vi "stirap_detect.vi"() -> ()   [LabVIEW 2012]
uses:
  <vilib>/DAQmx/create/channels.llb/DAQmx Create Channel (CO-Pulse Generation-Frequency).vi
  <vilib>/DAQmx/configure/timing.llb/DAQmx Timing (Implicit).vi
  <vilib>/Analysis/baseanly.llb/Mean (DBL).vi
  <vilib>/Utility/file.llb/Write To Spreadsheet File (DBL).vi
  <vilib>/Analysis/NI_AALBase.lvlib
panel:
  out "Fluorescence\n Mean Before":dbl format="%0.2f"
  in  "Save data to":path
  out "Fluorescence Before":T1(graph)
  out "Run Number":i32
  out "Total fluorescence with pumping":u32
  out "Total fluorescence without pumping":u32
  out "Optical pumping":bool
  out "Not_opt_pump_dark_runs":i32
  out "opt_pump_dark_runs":i32
  in  "Fluoresence Threshold":u32
  out "No_opt_pump_dark_run_ratio":dbl
  out "Opt_pump_Dark_run_ratio":dbl
  out "Fluorescence After":T2(graph)
  in  "Runs":i32
  in  "stop":bool
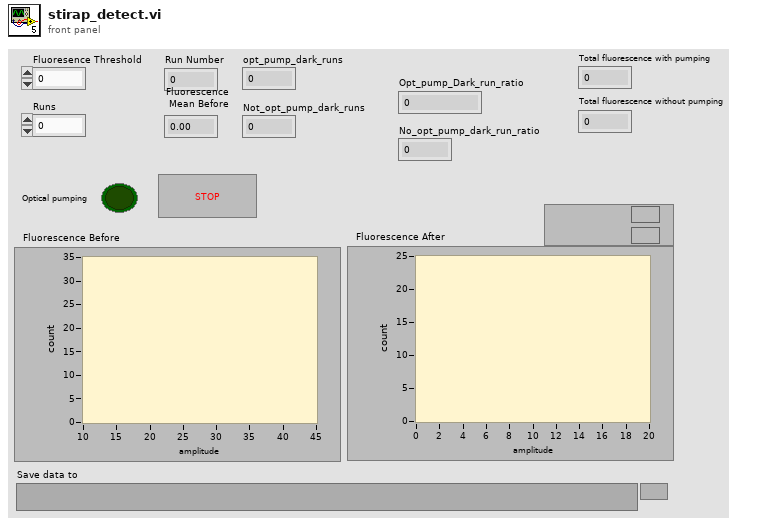
[diagram p1: front panel]
types:
  T1 = cluster{"X Values":dbl[], "Histogram: h(x)":i32[]}
  T2 = cluster{"X Values":dbl[], "Histogram: h(x)":i32[]}[]
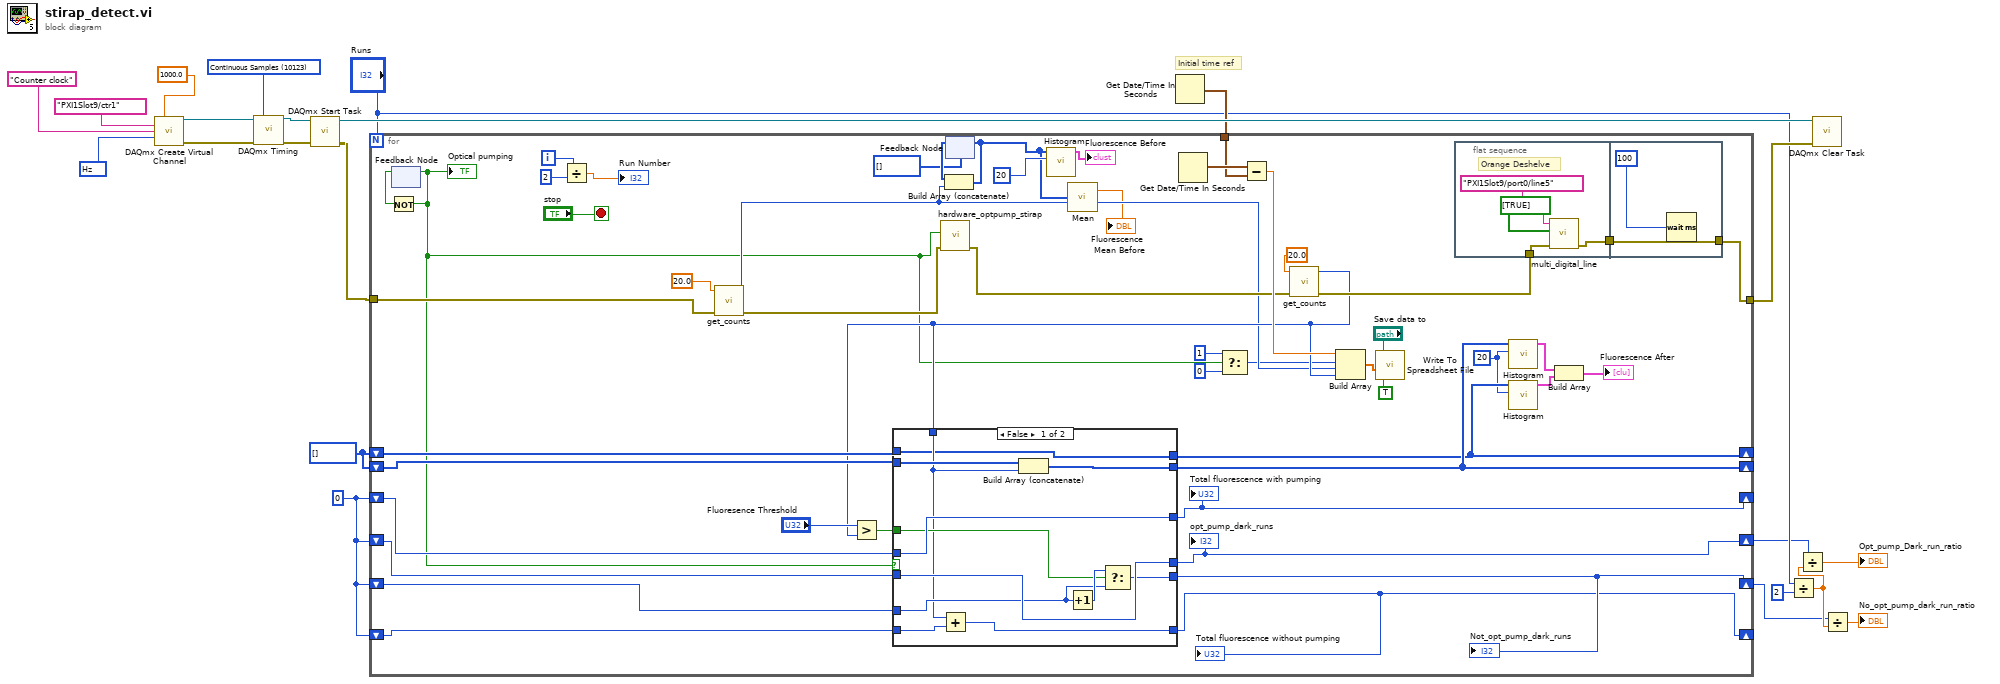
[diagram p0: block diagram]
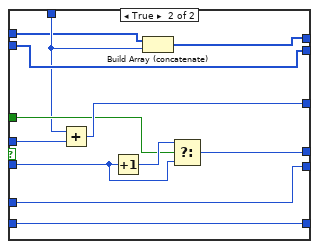
[diagram p2: hidden frame]
diagram:
  w2 = i32[] [] ("initialized array")
  w1 = 0
  w17 = 10123 items=["Finite Samples"=10178, "Continuous Samples"=10123, "Hardware Timed Single Point"=12522] ("sample mode")
  w22 = 10373 items=["Hz"=10373] ("units")
  # "Initial time ref"
  n1 = call-poly <vilib>:"DAQmx Create Virtual Channel.vi"("frequency"=1000.0 ("rate"), "counter"=tag "PXI1Slot9/ctr1", "name to assign"="Counter clock", "units"=w22) -> ("task out"=w21:refnum<k21>, "error out"=w20:errorcluster)  [unwired: 10 in]
  n2 = call-poly <vilib>:"DAQmx Timing.vi"("task/channels in"=w21, "sample mode"=w17, "error in"=w20) -> ("task out"=w19:refnum<k21>, "error out"=w18:errorcluster)  [unwired: 11 in]
  n3 = call <vilib>:"DAQmx Start Task.vi"("task/channels in"=w19, "error in"=w18) -> ("task out"=w12:refnum<k21>, "error out"=w13:errorcluster)  [unwired: 12 in]
  n4 = Get Date/Time In Seconds() -> (seconds since 1Jan1904=w11:timestamp)
  n5 = for {
    N: "Runs" -> [_]
    tunnel: w13 -> [w65]
    tunnel: w11 -> [w68]
    tunnel: [w61] -> w10
    shift-right: [w44] -> _
    shift-left: w2 -> [w45]
    shift-right: [w42] -> _
    shift-left: w2 -> [w43]
    shift-right: [w57] -> w5
    shift-left: w1 -> [w64]
    shift-right: [w56] -> w7
    shift-left: w1 -> [w63]
    shift-right: [w52] -> _
    shift-left: w1 -> [w54]
    shift-right: [w53] -> _
    shift-left: w1 -> [w55]
    i -> [w50]
    stop <- "stop" stop-if-true
    w41 = 20 ("intervals")
    n6 = feedback #1() -> (w48:bool)  [unwired: 1 in]
    n7 = Not(x=w48) -> (.not. x?=w32:bool)
    "Optical pumping" <- w32
    n8 = feedback-in #1(w32) -> ()
    n9 = Divide(x=w50, y=2) -> (x/y=→"Run Number":dbl)
    n10 = call "get_counts.vi"("error in"=w65, "Detection length (ms)"=20.0) -> ("error out"=w59:errorcluster, "Counts"=w33:u32)  [unwired: 8 in]
    n11 = call "hardware_optpump_stirap.vi"("error in"=w59, "Pump?"=w32) -> ("error out"=w58:errorcluster)  [unwired: 9 in]
    n12 = feedback #2(u32[] []) -> (w37:u32[])
    n13 = Build Array (concatenate)(w37, w33) -> (w24:u32[])
    n14 = feedback-in #2(w24) -> ()
    n15 = call <vilib>:"Histogram.vi"("intervals"=20, "X"=w24) -> ("Histogram Graph"=→"Fluorescence Before":T1)  [unwired: 6 in, 3 out]
    n16 = call-poly <vilib>:"Mean.vi"("X"=w24) -> ("mean"=→"Fluorescence\n Mean Before":dbl)  [unwired: 1 out]
    n17 = Get Date/Time In Seconds() -> (seconds since 1Jan1904=w69:timestamp)
    n18 = Select(t=1, s=w32, f=0) -> (s? t:f=w29:i32)
    n19 = Subtract(x=w69, y=w68) -> (x-y=w67:dbl)
    n20 = call "get_counts.vi"("error in"=w58, "Detection length (ms)"=20.0) -> ("error out"=w62:errorcluster, "Counts"=w34:u32)  [unwired: 8 in]
    n21 = Greater?(x="Fluoresence Threshold", y=w34) -> (0:w46:bool)
    n22 = case shown="False" w32 {
      tunnel: w64 -> [w84 w101]
      tunnel: w63 -> [w89 w96]
      tunnel: [w83 w101] -> w57
      tunnel: [w89 w95] -> w56
      tunnel: w34 -> [w80 w91]
      tunnel: w54 -> [w88 w100]
      tunnel: [w87 w100] -> w52
      tunnel: w55 -> [w86 w99]
      tunnel: [w86 w98] -> w53
      tunnel: w46 -> [w82 w94]
      tunnel: w45 -> [w81 w92]
      tunnel: [w79 w92] -> w44
      tunnel: [w78 w93] -> w42
      tunnel: w43 -> [w78 w90]
      frame False {
        n23 = Add(x=w80, y=w88) -> (x+y=w87:u32)
        n24 = Build Array (concatenate)(w81, w80) -> (w79:u32[])
        n25 = Increment(x=w84) -> (x+1=w85:i32)
        n26 = Select(t=w85, s=w82, f=w84) -> (s? t:f=w83:i32)
      }
      frame True {
        n27 = Add(x=w91, y=w99) -> (x+y=w98:u32)
        n28 = Increment(x=w96) -> (x+1=w97:i32)
        n29 = Build Array (concatenate)(w90, w91) -> (w93:u32[])
        n30 = Select(t=w97, s=w94, f=w96) -> (s? t:f=w95:i32)
      }
    }
    "opt_pump_dark_runs" <- w56
    "Not_opt_pump_dark_runs" <- w57
    "Total fluorescence with pumping" <- w53
    "Total fluorescence without pumping" <- w52
    n31 = Build Array(w67, w29, w33, w34) -> (w28:dbl[])
    n32 = call-poly <vilib>:"Write To Spreadsheet File.vi"("append to file? (new file:F)"=TRUE, "1D data"=w28, "file path (dialog if empty)"="Save data to") -> ()  [unwired: 5 in, 1 out]
    n33 = flat-sequence {
      tunnel: w62 -> [w75]
      tunnel: [w72] -> w60
      tunnel: [w77] -> w61
      tunnel: w60 -> [w77]
      frame #0 {
        # "Orange Deshelve"
        n34 = call "multi_digital_line.vi"("error in"=w75, "data"=bool[] [TRUE], "lines"=tag "PXI1Slot9/port0/line5" ("lines 2")) -> ("error out"=w72:errorcluster)  [unwired: 8 in]
      }
      frame #1 {
        n35 = Wait (ms)(milliseconds to wait=u32 100 ("455 Pumping Time 2")) -> ()  [unwired: 1 out]
      }
    }
    n36 = call <vilib>:"Histogram.vi"("intervals"=w41, "X"=w44) -> ("Histogram Graph"=w40:T1)  [unwired: 6 in, 3 out]
    n37 = call <vilib>:"Histogram.vi"("intervals"=w41, "X"=w42) -> ("Histogram Graph"=w39:T1)  [unwired: 6 in, 3 out]
    n38 = Build Array(w40, w39) -> (→"Fluorescence After":T2)
  }
  n39 = Divide(x="Runs", y=2) -> (x/y=w6:dbl)
  n40 = Divide(x=w7, y=w6) -> (x/y=→"Opt_pump_Dark_run_ratio":dbl)
  n41 = call <vilib>:"DAQmx Clear Task.vi"("task in"=w12, "error in"=w10) -> ()  [unwired: 13 in, 1 out]
  n42 = Divide(x=w5, y=w6) -> (x/y=→"No_opt_pump_dark_run_ratio":dbl)
